vi "_old_Comment_String_Expand.vi"(0 "Intial Comment String":string, 1 "Halt":bool) -> (2 "Option":T1(ring), 3 "Loops":u32, 4 "Marker String":string, 5 "Final Comment String":string)   [LabVIEW 2013]
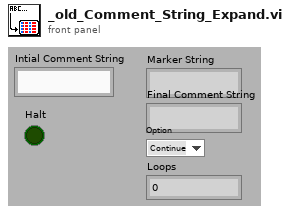
[diagram p1: front panel]
types:
  T1 = enum16{"Continue", "Ramp", "Loop", "EndLoop", "Halt"}
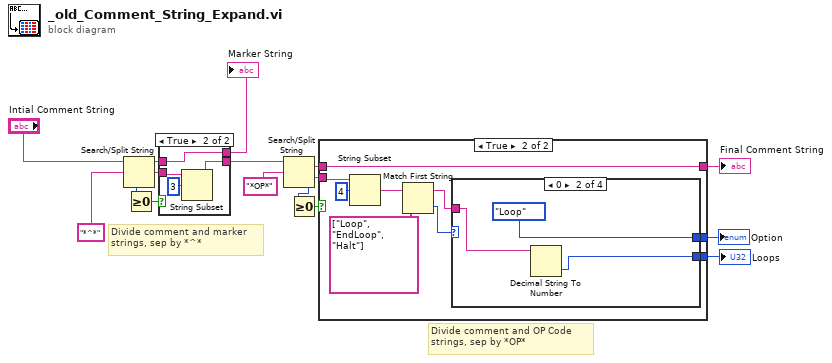
[diagram p0: block diagram]
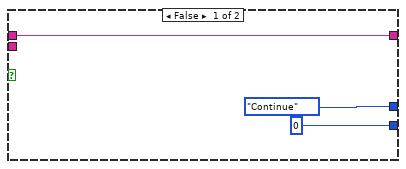
[diagram p2: hidden frame]
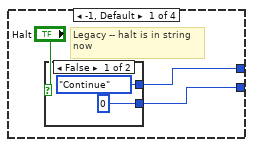
[diagram p3: hidden frame]
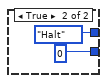
[diagram p4: hidden frame]
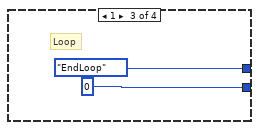
[diagram p5: hidden frame]
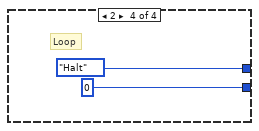
[diagram p6: hidden frame]
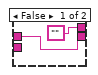
[diagram p7: hidden frame]
diagram:
  # "Divide comment and OP Code\nstrings, sep by *OP*"
  # "Divide comment and marker\nstrings, sep by *^*"
  n1 = Search/Split String(string="Intial Comment String", search string/char (-)="*^*") -> (substring before match=w12:string, match + rest of string=w15:string, offset of match=w14:i32)  [unwired: 1 out]
  n2 = Greater Or Equal To 0?(x=w14) -> (x >= 0?=w13:bool)
  n3 = case shown="True" w13 {
    tunnel: w15 -> [_ w22]
    tunnel: [w18 w20] -> w10
    tunnel: w12 -> [w18 w19]
    tunnel: ["" w19] -> w4
    frame False {
    }
    frame True {
      n4 = String Subset(string=w22, offset (0)=3) -> (substring=w20:string)  [unwired: 1 out]
    }
  }
  "Marker String" <- w4
  n5 = Search/Split String(string=w10, search string/char (-)="*OP*") -> (substring before match=w6:string, match + rest of string=w7:string, offset of match=w9:i32)  [unwired: 1 out]
  n6 = Greater Or Equal To 0?(x=w9) -> (x >= 0?=w8:bool)
  n7 = case shown="True" w8 {
    tunnel: w7 -> [_ w27]
    tunnel: [w25 w28] -> w3
    tunnel: w6 -> [w25 w28]
    tunnel: [T1."Continue" ("Option") w31] -> w2
    tunnel: [0 w30] -> w1
    frame False {
    }
    frame True {
      n8 = String Subset(string=w27, offset (0)=4) -> (substring=w26:string)  [unwired: 1 out]
      n9 = Match First String(2:string[] ["Loop", "EndLoop", "Halt"], 3:w26) -> (0:w32:i32, 1:w29:string)
      n10 = case shown="0" w32 {
        tunnel: [w37 T1."Loop" ("Option") T1."EndLoop" ("Option") T1."Halt" ("Option")] -> w31
        tunnel: [w36 w42 0 0] -> w30
        tunnel: w29 -> [_ w43 _ _]
        frame -1, Default {
          # "Legacy -- halt is in string\nnow"
          n11 = case shown="False" "Halt" {
            tunnel: [T1."Continue" ("Option") T1."Halt" ("Option")] -> w37
            tunnel: [0 0] -> w36
            frame False {
            }
            frame True {
            }
          }
        }
        frame 0 {
          n12 = Decimal String To Number(string=w43) -> (number=w42:i32)  [unwired: 3 out]
        }
        frame 1 {
          # "Loop"
        }
        frame 2 {
          # "Loop"
        }
      }
    }
  }
  "Final Comment String" <- w3
  "Loops" <- w1
  "Option" <- w2
